vi "ServoRpi.vi"() -> ()   [LabVIEW 2020]
uses:
  <vilib>/MakerHub/LINX/Public/Utilities/Open Serial.vi
  <vilib>/MakerHub/LINX/Public/Sensors/Motion/Servo/Servo Open One Channel.vi
  UnghiServoGlobal.vi
  <vilib>/MakerHub/LINX/Public/Sensors/Motion/Servo/Servo Set Pulse Width One Channel.vi
  <vilib>/MakerHub/LINX/Public/Sensors/Motion/Servo/Servo Close One Channel.vi
  <vilib>/MakerHub/LINX/LMH-LINX.lvlib
  <vilib>/Analysis/NI_AALPro.lvlib
  <vilib>/MakerHub/LINX/Public/Sensors/Motion/Servo/Servo.lvlib
panel:
  out "Servo":dbl=30.0
  in  "Meniu Input":T1(ring)
  in  "Unghi Servo":dbl(knob) min=0.0 max=165.0 step=5.0 scale=0.0..165.0
  in  "stop":bool
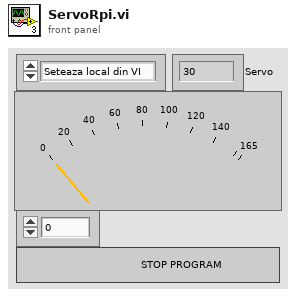
[diagram p1: front panel]
types:
  T1 = enum16{"Seteaza local din VI", "Seteaza din Web Service"}
  T2 = typedef "LMH-LINX.lvlib/LINX Ref.ctl" = cluster{"IO":T3, "Interface":T4, "LINX Device Config":T5}
  T3 = typedef "LMH-LINX.lvlib/Platform.ctl" = enum16{"Remote", "Local"}
  T4 = typedef "LMH-LINX.lvlib/Interface.ctl" = enum16{"Serial", "TCP"}
  T5 = typedef "LMH-LINX.lvlib/Device.lvlib/LINX Device Config.ctl" = cluster{"Interface":T4, "COM Port":refnum<visa-resource-name>, "TCP Configuration":T6, "Device Family":u8, "Device ID":u8, "Device Name":string, "TCP Ref":refnum<k5>, "Channels":T7}
  T6 = typedef "LMH-LINX.lvlib/Device.lvlib/TCP Config.ctl" = cluster{"IP Address":string, "Port":u16}
  T7 = typedef "LMH-LINX.lvlib/Channels.ctl" = cluster{"DI":u8[], "DO":u8[], "AI":u8[], "AO":u8[], "PWM":u8[], "QE":u8[], "UART":u8[], "I2C 2":u8[], "SPI":u8[], "CAN":u8[], "Servo":u8[], "AI Ref (V)":dbl, "AI Resolution (Bits)":u8, "AO Ref (V)":dbl, "AO Resolution (Bits)":u8}
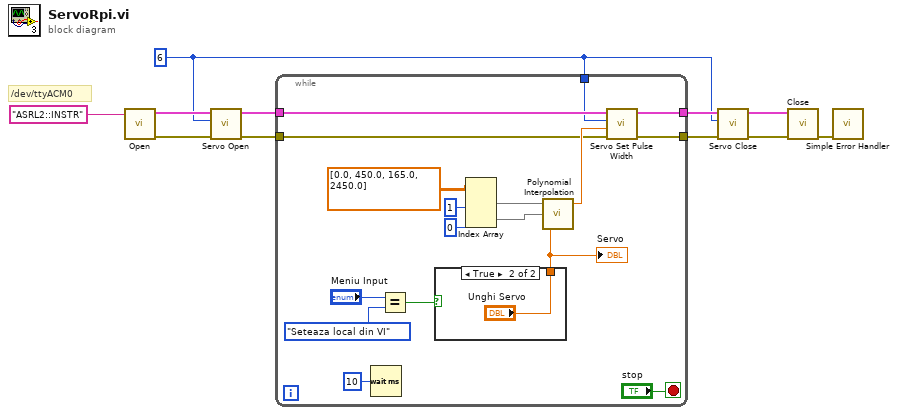
[diagram p0: block diagram]
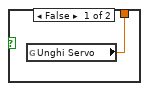
[diagram p2: hidden frame]
diagram:
  w2 = i8 6 ("Servo Channel")
  # "/dev/ttyACM0"
  n1 = call-poly <vilib>:"Open.vi"("Serial Port"="ASRL2::INSTR") -> ("Error Out"=w7:errorcluster, "LINX Resource"=w8:T2)  [unwired: 8 in, 1 out]
  n2 = call-poly <vilib>:"Servo Open.vi"("Error In"=w7, "Servo Channel"=w2, "LINX Resource"=w8) -> ("Error Out"=w9:errorcluster, "LINX Resource"=w10:T2)  [unwired: 7 in]
  n3 = while {
    tunnel: [w28] -> w6
    tunnel: [w27] -> w5
    tunnel: w2 -> [w16]
    tunnel: w10 -> [w18]
    tunnel: w9 -> [w17]
    stop <- "stop" stop-if-true
    n4 = Wait (ms)(milliseconds to wait=u32 10) -> ()  [unwired: 1 out]
    n5 = Equal?(x="Meniu Input", y=T1."Seteaza local din VI") -> (x = y?=w15:bool)
    n6 = case shown="True" w15 {
      tunnel: [w29 "Unghi Servo"] -> w12
      frame False {
        n7 = global read "UnghiServoGlobal.vi" "Unghi Servo"() -> (w29:dbl)
      }
      frame True {
      }
    }
    "Servo" <- w12
    n8 = Index Array(array=dbl[][] [[0.0, 450.0], [165.0, 2450.0]], index (col) #1=1 ("disabled index (col)"), index (col) #2=0 ("index (col)")) -> (element #1=w22:dbl[], element #2=w21:dbl[])  [unwired: 2 in]
    n9 = call <vilib>:"Polynomial Interpolation.vi"("x value"=w12, "X"=w21, "Y"=w22) -> ("interpolation value"=w24:dbl)  [unwired: 2 out]
    n10 = call-poly <vilib>:"Servo Set Pulse Width.vi"("Error In"=w17, "Pulse Width (uS)"=w24, "Servo Channel"=w16, "LINX Resource"=w18) -> ("Error Out"=w27:errorcluster, "LINX Resource"=w28:T2)  [unwired: 6 in]
  }
  n11 = call-poly <vilib>:"Servo Close.vi"("Error In"=w5, "Servo Channel"=w2, "LINX Resource"=w6) -> ("Error Out"=w3:errorcluster, "LINX Resource"=w4:T2)  [unwired: 7 in]
  n12 = call <vilib>:"Close.vi"("Error In"=w3, "LINX Resource"=w4) -> ("Error Out"=w11:errorcluster)  [unwired: 9 in]
  n13 = call <vilib>:"Simple Error Handler.vi"("error in (no error)"=w11) -> ()  [unwired: 4 in, 5 out]
